vi "String Default.vi"(5 "Default":string, 6 "String":string) -> (2 "String":string)   [LabVIEW 2017]
panel:
  # "Set string to default value if it is empty"
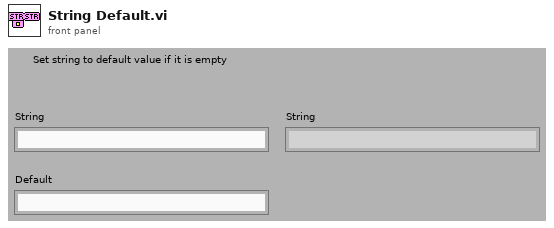
[diagram p1: front panel]
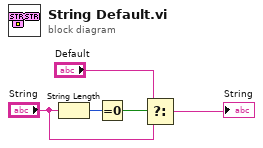
[diagram p0: block diagram]
diagram:
  n1 = String Length(string="String") -> (length=w5:i32)
  n2 = Equal To 0?(x=w5) -> (x = 0?=w4:bool)
  n3 = Select(t="Default", s=w4, f="String") -> (s? t:f=→"String":string)
